vi "Practica7.vi"() -> ()   [LabVIEW 2024]
uses:
  <vilib>/LabVIEW Interface for Arduino/Type Defs/Digital Pin.ctl
  <vilib>/LabVIEW Interface for Arduino/LabVIEW Interface for Arduino.lvlib
panel:
  in  "Digital Pin":T1
  in  "stop":bool
  in  "Boolean 2":bool
  out "Boolean":bool
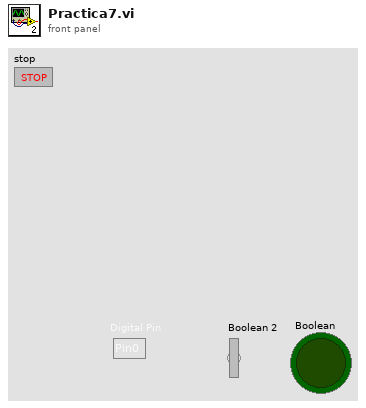
[diagram p1: front panel]
types:
  T1 = typedef "LabVIEW Interface for Arduino.lvlib/Digital Pin.ctl" = enum8{"Pin0", "Pin1", "Pin2", "Pin3", "Pin4", "Pin5", "Pin6", "Pin7", "Pin8", "Pin9", "Pin10", "Pin11", "Pin12", "Pin13"}
  T2 = typedef "LabVIEW Interface for Arduino.lvlib/Arduino Resource.ctl" = cluster{"VISA resource":refnum<visa-resource-name>, "Board Type":T3, "Connection Type":enum8{"USB / Serial"}, "Bytes Per Packet (15)":u8}
  T3 = typedef "LabVIEW Interface for Arduino.lvlib/Board Type.ctl" = enum16{"Uno", "Dimuelanove w/Atmega 328", "Mega 2560"}
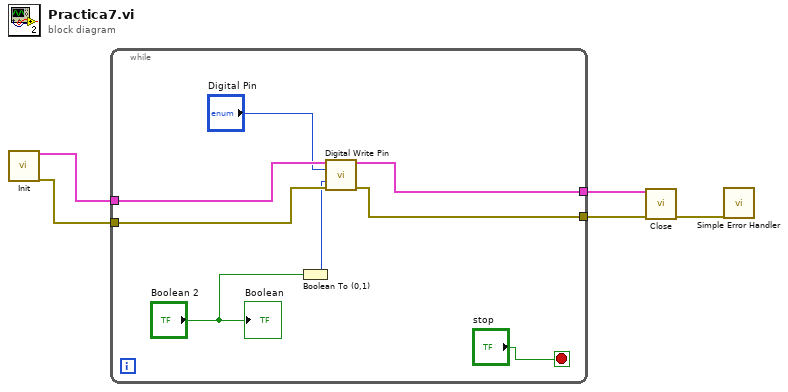
[diagram p0: block diagram]
diagram:
  n1 = call <vilib>:"Init.vi"() -> ("Arduino Resource"=w4:T2, "error out"=w3:errorcluster)  [unwired: 18 in]
  n2 = while {
    tunnel: w4 -> [w12]
    tunnel: w3 -> [w11]
    tunnel: [w10] -> w2
    tunnel: [w9] -> w1
    stop <- "stop" stop-if-true
    n3 = Boolean To (0,1)(Boolean="Boolean 2") -> (0, 1=w7:i16)
    n4 = call <vilib>:"Digital Write Pin.vi"("Arduino Resource"=w12, "Digital I/O Pin (0)"="Digital Pin", "Value (0)"=w7, "error in"=w11) -> ("Arduino Resource"=w9:T2, "error out"=w10:errorcluster)  [unwired: 10 in]
    "Boolean" <- "Boolean 2"
  }
  n5 = call <vilib>:"Close.vi"("Arduino Resource"=w1, "error in"=w2) -> ("error out"=w5:errorcluster)  [unwired: 13 in]
  n6 = call <vilib>:"Simple Error Handler.vi"("error in (no error)"=w5) -> ()  [unwired: 4 in, 5 out]
